vi "read_attributes.vi"(8 "error in (no error)":errorcluster, 11 "ExtraTreeRegressor in":refnum<class "ExtraTreeRegressor.lvclass">) -> (0 "error out":errorcluster, 2 "attributes":T1, 3 "ExtraTreeRegressor out":refnum<class "ExtraTreeRegressor.lvclass">)   [LabVIEW 2020, in "ExtraTreeRegressor.lvclass"]
uses:
  ExtraTreeRegressor.lvclass
  Controls/extra_tree_regressor_attributes.ctl
  ExtraTreeRegressor.lvclass/ExtraTreeRegressor.ctl
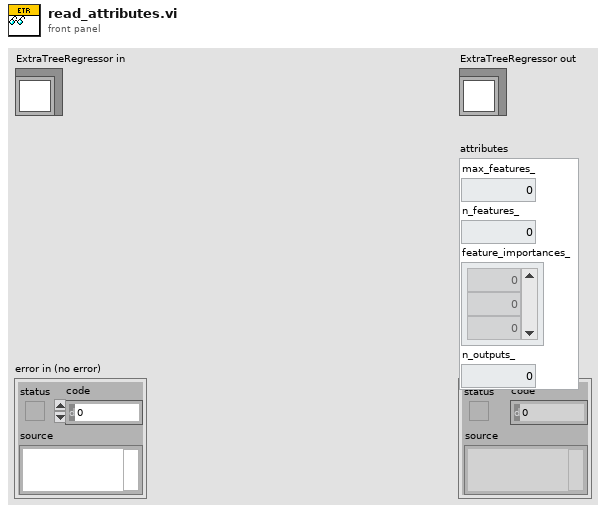
[diagram p1: front panel]
types:
  T1 = typedef "extra_tree_regressor_attributes.ctl" = cluster{"max_features_":dbl, "n_features_":dbl, "feature_importances_":dbl[], "n_outputs_":dbl}
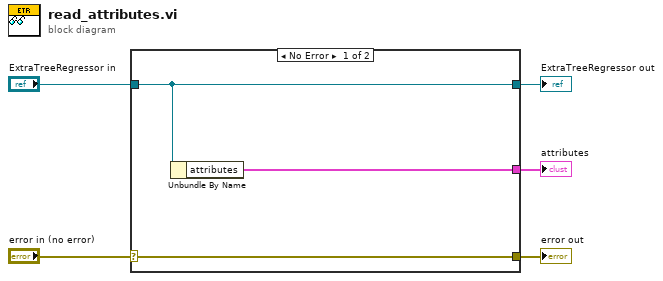
[diagram p0: block diagram]
diagram:
  n1 = case shown="No Error" "error in (no error)" {
    selector: "error in (no error)" -> [w8 w9]
    tunnel: [w8 w9] -> w4
    tunnel: [w7 w10] -> w2
    tunnel: "ExtraTreeRegressor in" -> [w7 w10]
    tunnel: [w6 _] -> w1
    frame No Error {
      n2 = Unbundle By Name(w7) -> ("attributes"=w6:T1)
    }
    frame Error {
    }
  }
  "error out" <- w4
  "ExtraTreeRegressor out" <- w2
  "attributes" <- w1
